vi "C843Config.vi"(0 "Limit Switch  Refnum":refnum<vi>, 1 "Axes to move Refnum":refnum<vi>, 2 "Initialisation OK Refnum":refnum<vi>, 3 "All Axes? Refnum":refnum<vi>, 4 "Stage names Input Refnum":refnum<vi>, 5 "Identification Refnum":refnum<vi>, 6 "Connected Axes Refnum":refnum<vi>, 7 "Position Refnum":refnum<vi>, 10 "+/- movement range Refnum":refnum<vi>, 11 "Error Out Refnum":refnum<vi>, 12 "LED status Refnum":refnum<vi>, 13 "Etat moteurs Refnum":refnum<vi>) -> ()   [LabVIEW 2013]
panel:
  out "Identification":string
  out "Conn. \nAxes":string[](array[string])
  out "Position":dbl[](array[numeric]) format="%.6f"
  out "+/- movement\nrange":dbl[](array[numeric]) format="%.6f"
  out "Stage names input":string[](array[string])
  out "All Axes?":bool
  out "Axes to Move":string[](array[string])
  out "Limit Switch":u16
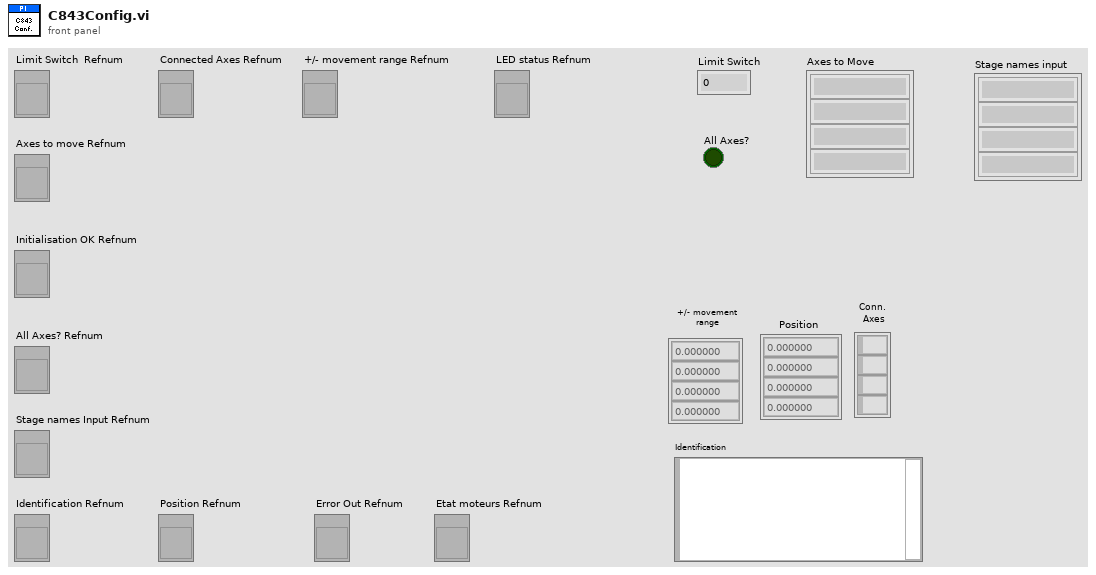
[diagram p1: front panel]
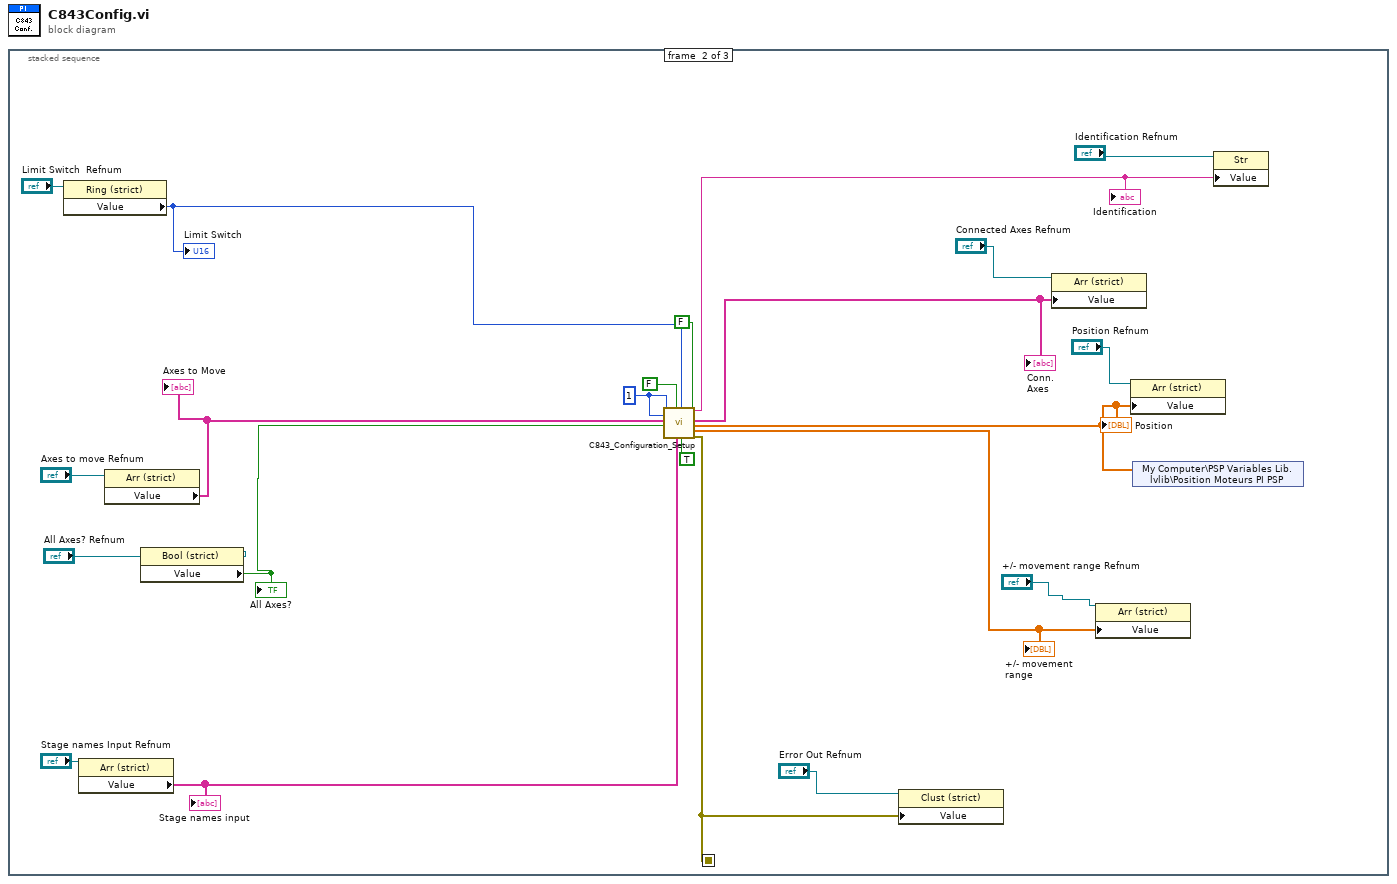
[diagram p0: block diagram]
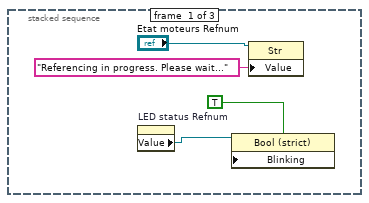
[diagram p2: hidden frame]
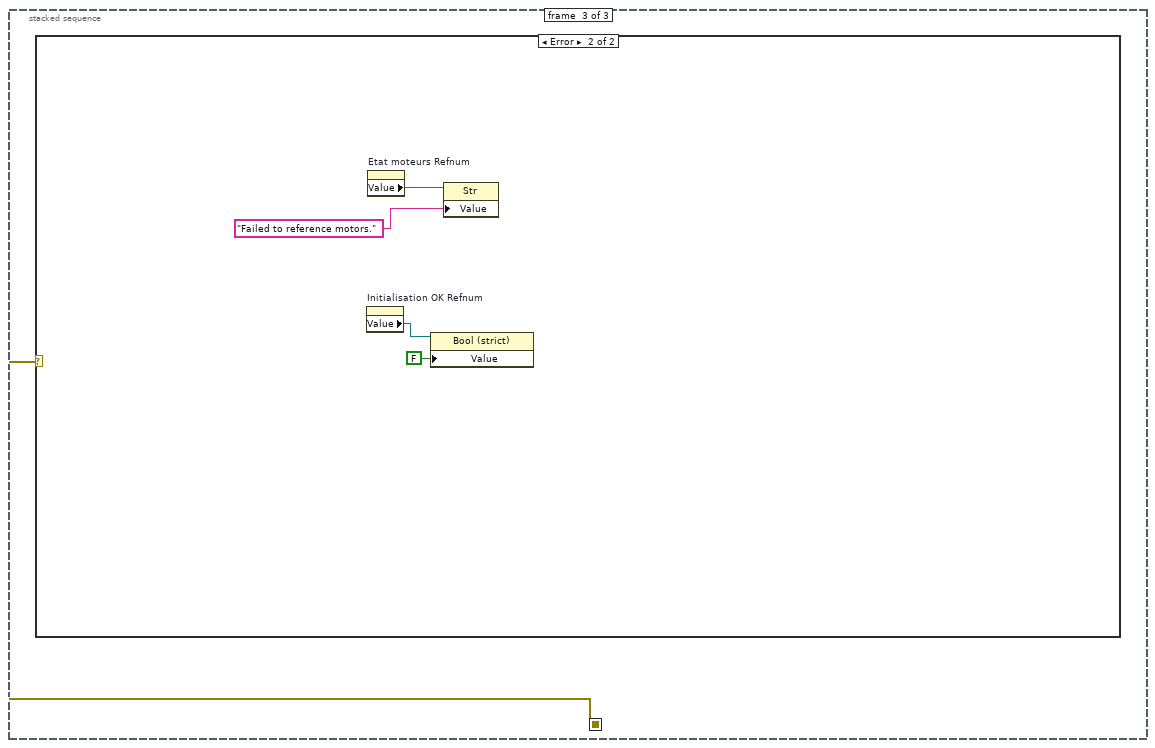
[diagram p3: hidden frame]
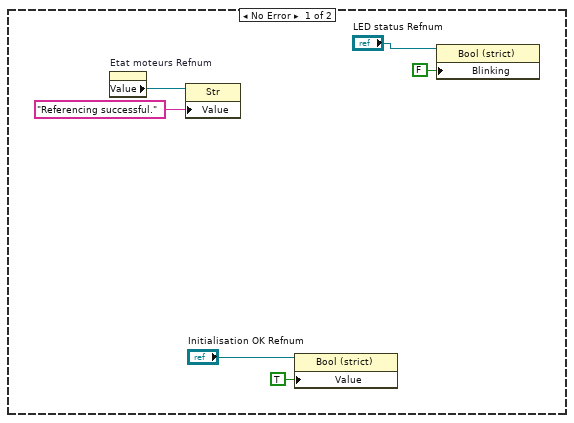
[diagram p4: hidden frame]
diagram:
  n1 = stacked-sequence {
    seq-local: [_ w11 _] -> [_ _ w27]
    frame #0 {
      n2 = property on="LED status Refnum" class="LVObjRef (strict)"() -> ("Value"=w2:refnum<vi>)  [unwired: 2 in, 2 out]
      n3 = property class="Bool (strict)"(reference=w2, "Blinking"=TRUE) -> ()  [unwired: 1 in, 2 out]
      n4 = property class="Str"(reference="Etat moteurs Refnum", "Value"="Referencing in progress. Please wait...") -> ()  [unwired: 1 in, 2 out]
    }
    frame #1 {
      w7 = 1 ("System no.")
      n5 = property class="Ring (strict)"(reference="Limit Switch  Refnum") -> ("Value"=w24:u16)  [unwired: 1 in, 2 out]
      "Limit Switch" <- w24
      n6 = property class="Arr (strict)"(reference="Stage names Input Refnum") -> ("Value"=w25:string[])  [unwired: 1 in, 2 out]
      "Stage names input" <- w25
      n7 = property class="Arr (strict)"(reference="Axes to move Refnum") -> ("Value"=w6:string[])  [unwired: 1 in, 2 out]
      "Axes to Move" <- w6
      n8 = property class="Bool (strict)"(reference="All Axes? Refnum") -> ("Value"=w26:bool)  [unwired: 1 in, 2 out]
      "All Axes?" <- w26
      n9 = call "C843_Configuration_Setup.vi"("System no."=w7, "C-843 Board No."=w7, "Axes to move"=w6, "All axes?"=w26, "Use dialog to define\nconnected stages?"=FALSE ("Use dialog to define\nconnected stages?"), "Stage names input"=w25, "Limit switch selection"=w24, "Define home?"=TRUE, "Move to middle?"=FALSE) -> ("Identification"=w23:string, "Conn. \nAxes"=w22:string[], "Position"=w10:dbl[], "+/- movement\nrange"=w21:dbl[], "error out"=w11:errorcluster)  [unwired: 6 in]
      "+/- movement\nrange" <- w21
      "Position" <- w10
      "Conn. \nAxes" <- w22
      "Identification" <- w23
      n10 = property class="Clust (strict)"(reference="Error Out Refnum", "Value"=w11) -> ()  [unwired: 1 in, 2 out]
      n11 = property class="Arr (strict)"(reference="Connected Axes Refnum", "Value"=w22) -> ()  [unwired: 1 in, 2 out]
      n12 = property class="Arr (strict)"(reference="+/- movement range Refnum", "Value"=w21) -> ()  [unwired: 1 in, 2 out]
      n13 = property class="Arr (strict)"(reference="Position Refnum", "Value"=w10) -> ()  [unwired: 1 in, 2 out]
      n14 = shared-variable "My Computer\\PSP Variables Lib.lvlib\\Position Moteurs PI PSP"(w10) -> ()  [unwired: 1 in, 1 out]
      n15 = property class="Str"(reference="Identification Refnum", "Value"=w23) -> ()  [unwired: 1 in, 2 out]
    }
    frame #2 {
      n16 = case shown="Error" w27 {
        frame No Error {
          n17 = property on="Etat moteurs Refnum" class="LVObjRef (strict)"() -> ("Value"=w33:refnum<vi>)  [unwired: 2 in, 2 out]
          n18 = property class="Str"(reference=w33, "Value"="Referencing successful.") -> ()  [unwired: 1 in, 2 out]
          n19 = property class="Bool (strict)"(reference="Initialisation OK Refnum", "Value"=TRUE) -> ()  [unwired: 1 in, 2 out]
          n20 = property class="Bool (strict)"(reference="LED status Refnum", "Blinking"=FALSE) -> ()  [unwired: 1 in, 2 out]
        }
        frame Error {
          n21 = property on="Initialisation OK Refnum" class="LVObjRef (strict)"() -> ("Value"=w35:refnum<vi>)  [unwired: 2 in, 2 out]
          n22 = property on="Etat moteurs Refnum" class="LVObjRef (strict)"() -> ("Value"=w37:refnum<vi>)  [unwired: 2 in, 2 out]
          n23 = property class="Bool (strict)"(reference=w35, "Value"=FALSE) -> ()  [unwired: 1 in, 2 out]
          n24 = property class="Str"(reference=w37, "Value"="Failed to reference motors.") -> ()  [unwired: 1 in, 2 out]
        }
      }
    }
  }
